vi "打开指定文件(8.0).vi"   [LabVIEW 2013]
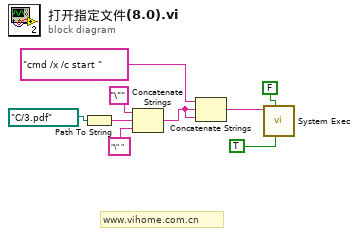
[diagram p0: block diagram]
diagram:
  # "www.vihome.com.cn"
  n1 = Path To String(path=path "C:/3.pdf" ("file name and path")) -> (string=w4:string)
  n2 = Concatenate Strings("\"" ("Substring"), w4, "\" " ("Substring")) -> (w3:string)
  n3 = Concatenate Strings("cmd /x /c start ", w3, w3) -> (w7:string)
  n4 = call <vilib>:"System Exec.vi"("run minimized? (F)"=TRUE, "wait until completion? (T)"=FALSE ("Wait until done"), "command line"=w7) -> ()  [unwired: 5 in, 4 out]
